vi "testAssertSourceSeparatedFromCompiledCodeReturnsExpected.vi"(8 "error in":errorcluster, 11 "TestCase in":refnum<class "VeriStandTestUtilitiesTests.lvclass">) -> (0 "error out":errorcluster, 3 "TestCase out":refnum<class "VeriStandTestUtilitiesTests.lvclass">)   [LabVIEW 2027, in "VeriStandTestUtilitiesTests.lvclass"]
uses:
  VeriStandTestUtilitiesTests.lvclass
  <vilib>/addons/_JKI Toolkits/VI Tester/TestCase.llb/TestCase.lvclass
  Source/VeriStandTestUtilities/VeriStandTestUtilities.lvlib
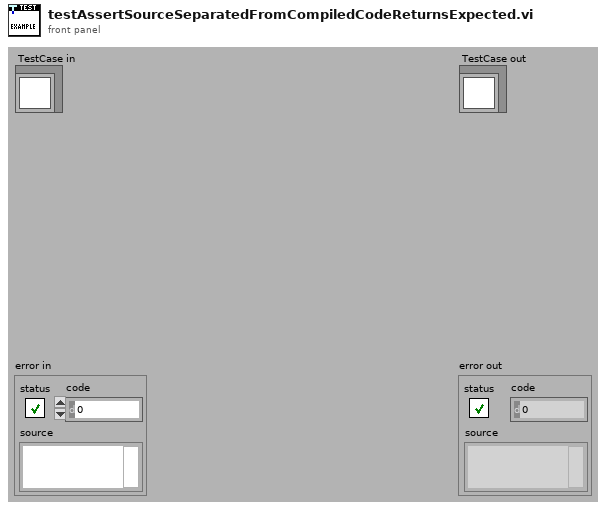
[diagram p1: front panel]
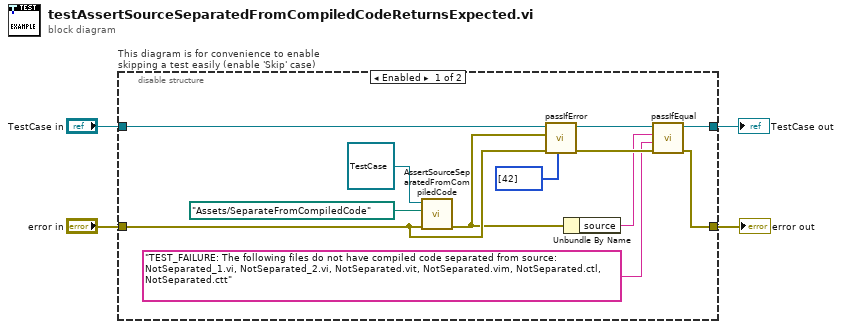
[diagram p0: block diagram]
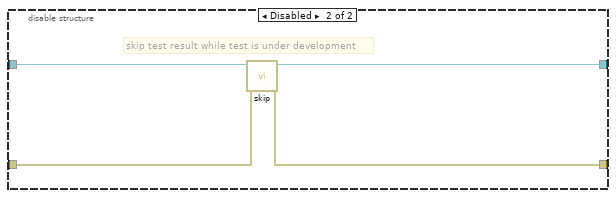
[diagram p2: hidden frame]
diagram:
  n1 = disable-structure "This diagram is for convenience to enable skipping a test easily (enable 'Skip' case)" shown="Enabled" {
    disable-tunnel: "TestCase in" -> [w13 w20]
    disable-tunnel: [w8 w18] -> w1
    disable-tunnel: [w10 w19] -> w3
    disable-tunnel: "error in" -> [w14 w17]
    frame Enabled {
      n2 = call "AssertSourceSeparatedFromCompiledCode.vi"("error in"=w14, "search path"=path "Assets/SeparateFromCompiledCode", "TestCase in"=refnum<class "TestCase.lvclass"> refnum) -> ("error out"=w7:errorcluster)  [unwired: 7 in, 1 out]
      n3 = call-dynamic "passIfError.vi"("passing error codes (default = any error code)"=i32[] [42], "error in (no error)"=w14, "error"=w7, "TestCase in"=w13) -> ("error out"=w11:errorcluster, "TestCase out"=w9:refnum<class "VeriStandTestUtilitiesTests.lvclass">)  [unwired: 6 in]
      n4 = Unbundle By Name(w7) -> ("source"=w6:string)
      n5 = call-dynamic "passIfEqual.vi"("error in (no error)"=w11, "y"="TEST_FAILURE: The following files do not have compiled code separated from source: NotSeparated_1.vi, NotSeparated_2.vi, NotSeparated.vit, NotSeparated.vim, NotSeparated.ctl, NotSeparated.ctt", "x"=w6, "TestCase in"=w9) -> ("error out"=w10:errorcluster, "TestCase out"=w8:refnum<class "VeriStandTestUtilitiesTests.lvclass">)  [unwired: 6 in]
    }
    frame Disabled {
      # "skip test result while test is under development"
      n6 = call <vilib>:"skip.vi"("error in (no error)"=w17, "TestCase in"=w20) -> ("error out"=w19:errorcluster, "TestCase out"=w18:refnum<class "VeriStandTestUtilitiesTests.lvclass">)  [unwired: 8 in]
    }
  }
  "error out" <- w3
  "TestCase out" <- w1
